vi "1 Tap 12-Bit.vi"() -> (0 "PixelData":u16)   [LabVIEW 2014]
uses:
  <vilib>/rvi/eio/common/nirviEmuTemplateMethod_errors.vi
  <vilib>/eio/EIONode/EIONode.xnode
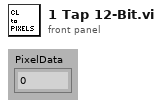
[diagram p1: front panel]
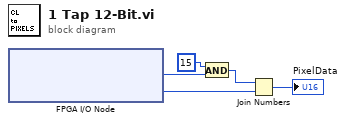
[diagram p0: block diagram]
diagram:
  n1 = xnode "FPGA I/O Node"() -> ("IO Module\\CL Port B"=w3:u8, "IO Module\\CL Port A"=w2:u8)  [unwired: 2 in, 2 out]
  n2 = And(x=u8 15 ("hi"), y=w3) -> (x .and. y?=w4:u8)
  n3 = Join Numbers(hi=w4, lo=w2) -> ((hi.lo)=→"PixelData":u16)
